vi "random_access_read.vi"(4 "ra scanning?":bool, 6 "ra trajectory pixels (data/pixels transfered)":u32=65535, 7 "FPGA parameters in":T3 {"AOD center frequ. (Hz)_y" format="%.14g"; "AOD half bandwidth_y" format="%.14g"; "AOD Bandwidth_y (Hz)" format="%_6f"; "AOD center frequ. (Hz)_x" format="%.14g"; "cos Phi" format="%.35g"; "sin Phi" format="%.35g"; "AOD_Scale_Factor (1/Zoom)" format="%.35g"; "AOD half bandwidth_x" format="%.14g"; "AOD Bandwidth_x (Hz)" format="%_6f"}, 8 "rotation cluster in":T1={"ellipsoid"={"counter"=0, "~x n"=0.999969482421875, "~y n"=0.0, "~z n"=5.0, "amp 0"=0.0}} {"ellipsoid"."amp 0" format="%.16g"; "ellipsoid"."~z n" format="%.11g"; "ellipsoid"."~y n" format="%.16g"; "ellipsoid"."~x n" format="%.16g"}, 10 "sub-pattern iterations per pixel":u16, 11 "scan points cluster in":T2) -> (0 "rotation cluster out":T1={"ellipsoid"={"counter"=0, "~x n"=0.999969482421875, "~y n"=0.0, "~z n"=5.0, "amp 0"=0.0}} {"ellipsoid"."amp 0" format="%.16g"; "ellipsoid"."~z n" format="%.11g"; "ellipsoid"."~y n" format="%.16g"; "ellipsoid"."~x n" format="%.16g"}, 2 "new pixel update?":bool, 3 "scan points cluster out":T2, 5 "FPGA parameters out":T3 {"AOD center frequ. (Hz)_y" format="%.14g"; "AOD half bandwidth_y" format="%.14g"; "AOD Bandwidth_y (Hz)" format="%_6f"; "AOD center frequ. (Hz)_x" format="%.14g"; "cos Phi" format="%.35g"; "sin Phi" format="%.35g"; "AOD_Scale_Factor (1/Zoom)" format="%.35g"; "AOD half bandwidth_x" format="%.14g"; "AOD Bandwidth_x (Hz)" format="%_6f"})   [LabVIEW 2010]
uses:
  FPGA_parameters_cluster.ctl
  scan_points_cluster.ctl
  anti-photo-bleaching_rotation_cluster.ctl
  <vilib>/rvi/DataTransferAndStorage/Container/XNode/niFpgaContainer.xnode
  <vilib>/rvi/FIFO/Fifo_Resource/nirvififoEmulationSetSize.vi
  <vilib>/rvi/DataTransferAndStorage/Container/Common/niFpgaContainerGetUniqueNameForEmu.vi
  <vilib>/rvi/Memory/Memory_Emulation/nirvimemoryEmulationManagerCache_GetValue.vi
  <vilib>/rvi/Memory/Memory_Emulation/nirvimemoryEmulationManagerCache_InsertValue.vi
  <vilib>/Utility/error.llb/Clear Errors.vi
  <vilib>/rvi/Memory/Memory_Emulation/nirvimemoryEmulationManagerCache_SetValue.vi
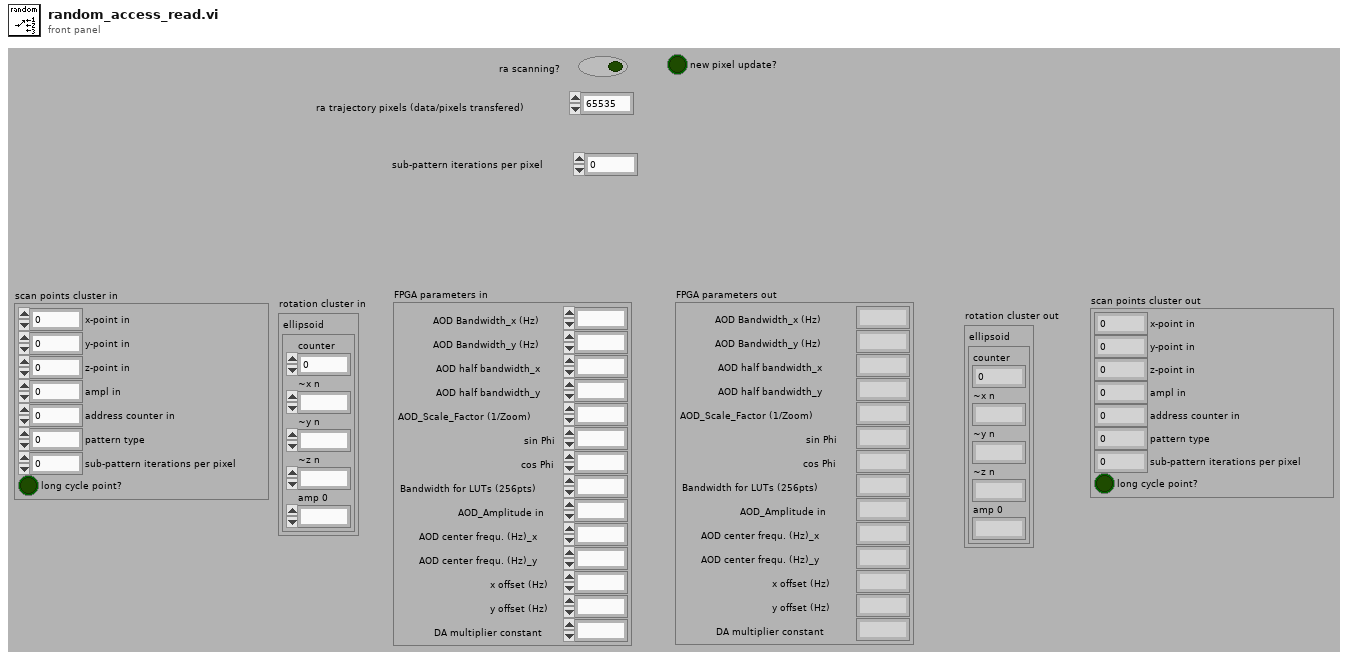
[diagram p1: front panel]
types:
  T1 = typedef "anti-photo-bleaching_rotation_cluster.ctl" = cluster{"ellipsoid":cluster{"counter":u16, "~x n":fxp<+/-,16,1>, "~y n":fxp<+/-,16,1>, "~z n":fxp<+/-,16,8>, "amp 0":fxp<+/-,16,1>}}
  T2 = typedef "scan_points_cluster.ctl" = cluster{"x-point in":u16, "y-point in":u16, "z-point in":u16, "ampl in":u16, "address counter in":i32, "pattern type":i8, "sub-pattern iterations per pixel":u16, "long cycle point?":bool}
  T3 = typedef "FPGA_parameters_cluster.ctl" = cluster{"AOD Bandwidth_x (Hz)":fxp<+,36,32>, "AOD Bandwidth_y (Hz)":fxp<+,36,32>, "AOD half bandwidth_x":fxp<+,36,32>, "AOD half bandwidth_y":fxp<+,36,32>, "AOD_Scale_Factor (1/Zoom)":fxp<+,36,2>, "sin Phi":fxp<+/-,36,2>, "cos Phi":fxp<+/-,36,2>, "Bandwidth for LUTs (256pts)":fxp<+,36,0>, "AOD_Amplitude in":u16, "AOD center frequ. (Hz)_x":fxp<+,36,32>, "AOD center frequ. (Hz)_y":fxp<+,36,32>, "x offset (Hz)":fxp<+/-,36,32>, "y offset (Hz)":fxp<+/-,36,32>, "DA multiplier constant":fxp<+,64,4>}
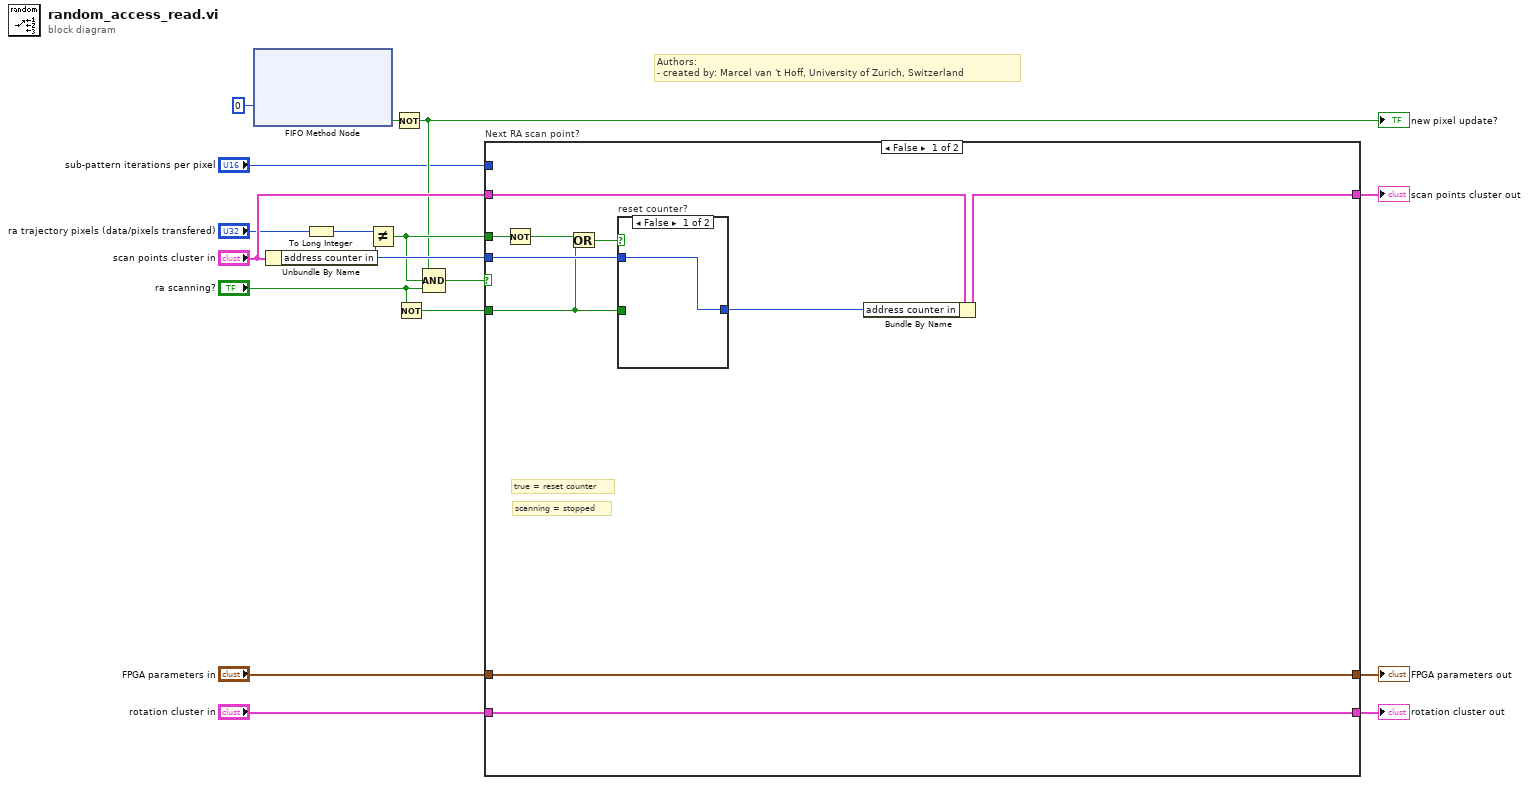
[diagram p0: block diagram]
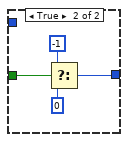
[diagram p2: hidden frame]
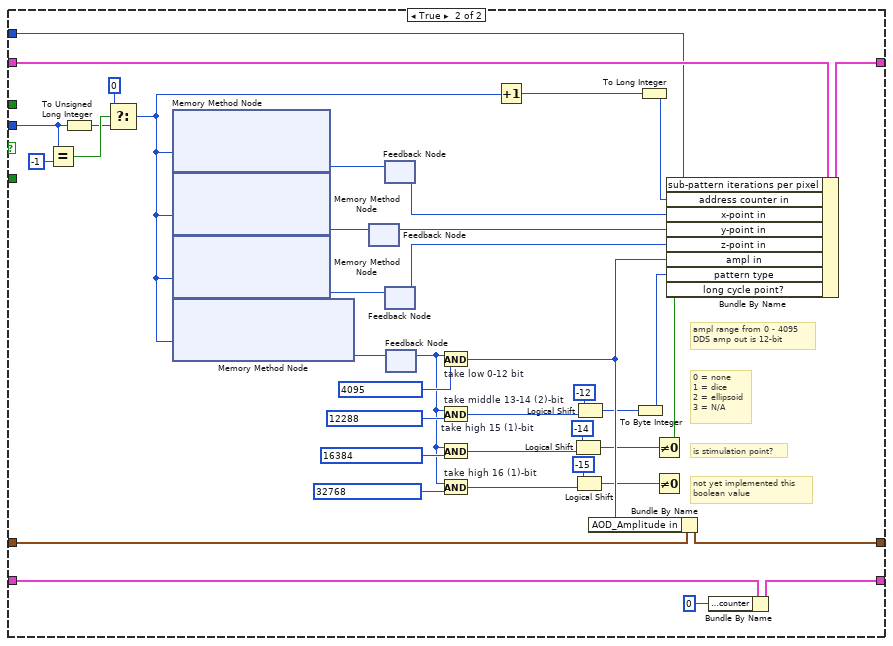
[diagram p3: hidden frame]
diagram:
  # "Authors: \n- created by: Marcel van 't Hoff, University of Zurich, Switzerland"
  n1 = xnode ("FIFO Method Node")("Timeout"=0) -> ("Timed Out?"=w16:bool)  [unwired: 1 in, 2 out]
  n2 = Unbundle By Name("scan points cluster in") -> ("address counter in"=w10:i32)
  n3 = To Long Integer(number="ra trajectory pixels (data/pixels transfered)") -> (32bit integer=w4:i32)
  n4 = Not Equal?(x=w4, y=w10) -> (x != y?=w8:bool)
  n5 = Not(x=w16) -> (.not. x?=w7:bool)
  "new pixel update?" <- w7
  n6 = Not(x="ra scanning?") -> (.not. x?=w14:bool)
  n7 = Compound Arithmetic op=AND(w7, w8, "ra scanning?") -> (w15:bool)
  n8 = case "Next RA scan point?" shown="False" w15 {
    tunnel: w14 -> [w19 _]
    tunnel: w10 -> [w20 w59]
    tunnel: w8 -> [w27 _]
    tunnel: "FPGA parameters in" -> [w26 w72]
    tunnel: [w26 w71] -> w12
    tunnel: [w22 w66] -> w6
    tunnel: "scan points cluster in" -> [w23 w63]
    tunnel: [w18 w35] -> w3
    tunnel: "rotation cluster in" -> [w18 w36]
    tunnel: "sub-pattern iterations per pixel" -> [_ w33]
    frame False {
      # "scanning = stopped"
      # "true = reset counter"
      n9 = Not(x=w27) -> (.not. x?=w21:bool)
      n10 = Or(x=w21, y=w19) -> (x .or. y?=w25:bool)
      n11 = case "reset counter?" shown="False" w25 {
        tunnel: [w28 w29] -> w24
        tunnel: w20 -> [w28 _]
        tunnel: w19 -> [_ w32]
        frame False {
        }
        frame True {
          n12 = Select(t=-1 ("counter in"), s=w32, f=0 ("counter in")) -> (s? t:f=w29:i32)
        }
      }
      n13 = Bundle By Name(cluster=w23, "address counter in"=w24) -> (w22:T2)
    }
    frame True {
      # "is stimulation point?"
      # "not yet implemented this\nboolean value"
      # "0 = none\n1 = dice\n2 = ellipsoid\n3 = N/A"
      # "ampl range from 0 - 4095\nDDS amp out is 12-bit"
      n14 = Equal?(x=w59, y=-1) -> (x = y?=w60:bool)
      n15 = To Unsigned Long Integer(number=w59) -> (unsigned 32bit integer=w56:u32)
      n16 = Select(t=u32 0, s=w60, f=w56) -> (s? t:f=w57:u32)
      n17 = xnode ("Memory Method Node")("Address"=w57) -> ("Data"=w68:u16)  [unwired: 1 in, 1 out]
      n18 = xnode ("Memory Method Node")("Address"=w57) -> ("Data"=w69:u16)  [unwired: 1 in, 1 out]
      n19 = xnode ("Memory Method Node")("Address"=w57) -> ("Data"=w70:u16)  [unwired: 1 in, 1 out]
      n20 = xnode ("Memory Method Node")("Address"=w57) -> ("Data"=w51:u16)  [unwired: 1 in, 1 out]
      n21 = feedback #1() -> (w65:u16)  [unwired: 1 in]
      n22 = feedback-in #1(w69) -> ()
      n23 = feedback #2() -> (w67:u16)  [unwired: 1 in]
      n24 = feedback-in #2(w68) -> ()
      n25 = feedback #3() -> (w64:u16)  [unwired: 1 in]
      n26 = feedback-in #3(w70) -> ()
      n27 = feedback #4() -> (w48:u16)  [unwired: 1 in]
      n28 = feedback-in #4(w51) -> ()
      n29 = And "take low 0-12 bit"(x=w48, y=u16 4095) -> (x .and. y?=w52:u16)
      n30 = And "take middle 13-14 (2)-bit"(x=w48, y=u16 12288) -> (x .and. y?=w45:u16)
      n31 = And "take high 15 (1)-bit"(x=w48, y=u16 16384) -> (x .and. y?=w41:u16)
      n32 = And "take high 16 (1)-bit"(x=w48, y=u16 32768) -> (x .and. y?=w37:u16)
      n33 = Increment(x=w57) -> (x+1=w62:u32)
      n34 = Logical Shift(y=i16 -14, x=w41) -> (x << y=w40:u16)
      n35 = Logical Shift(y=i16 -15, x=w37) -> (x << y=w38:u16)
      n36 = Logical Shift(y=i16 -12, x=w45) -> (x << y=w44:u16)
      n37 = Bundle By Name(cluster=w72, "AOD_Amplitude in"=w52) -> (w71:T3)
      n38 = To Byte Integer(number=w44) -> (8bit integer=w43:i8)
      n39 = To Long Integer(number=w62) -> (32bit integer=w55:i32)
      n40 = Not Equal To 0?(x=w40) -> (x != 0?=w47:bool)
      n41 = Not Equal To 0?(x=w38) -> ()  [unwired: 1 out]
      n42 = Bundle By Name(cluster=w63, "sub-pattern iterations per pixel"=w33, "address counter in"=w55, "x-point in"=w67, "y-point in"=w65, "z-point in"=w64, "ampl in"=w52, "pattern type"=w43, "long cycle point?"=w47) -> (w66:T2)
      n43 = Bundle By Name(cluster=w36, "ellipsoid.counter"=u16 0) -> (w35:T1)
    }
  }
  "FPGA parameters out" <- w12
  "scan points cluster out" <- w6
  "rotation cluster out" <- w3
